vi "Query Element Type.vi"(8 "error in (no error)":errorcluster, 11 "VISA resource name":refnum<visa-resource-name>) -> (0 "error out":errorcluster, 2 "Element Type":i32[](array[numeric]), 3 "VISA resource name out":refnum<visa-resource-name>)   [LabVIEW 2021, in "Yokogawa WT1800 Series.lvlib"]
doc: "Queries the current instrument element type."
uses:
  <instrlib>/Yokogawa WT1800 Series/Yokogawa WT1800 Series.lvlib
panel:
  # "Element 1"
  # "Element 2"
  # "Element 3"
  # "Element 4"
  # "Element 5"
  # "Element 6"
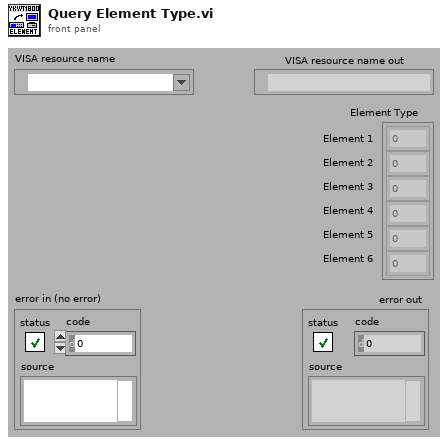
[diagram p1: front panel]
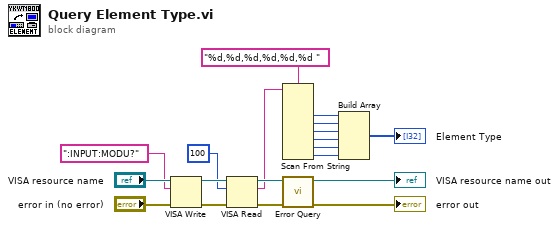
[diagram p0: block diagram]
diagram:
  n1 = VISA Write ("VISA書き込み")(VISA resource name="VISA resource name", write buffer=":INPUT:MODU?" ("書き込みバッファ"), error in (no error)="error in (no error)") -> (VISA resource name out=w19:refnum<visa-resource-name>, error out=w18:errorcluster)  [unwired: 1 out]
  n2 = VISA Read ("VISA読み取り")(VISA resource name=w19, byte count=u32 100, error in (no error)=w18) -> (VISA resource name out=w16:refnum<visa-resource-name>, read buffer=w9:string, error out=w14:errorcluster)  [unwired: 1 out]
  n3 = Scan From String(format string="%d,%d,%d,%d,%d,%d " ("形式文字列"), input string=w9) -> (output 1=w7:i32, output 2=w6:i32, output 3=w5:i32, output 4=w4:i32, output 5=w3:i32, output 6=w2:i32)  [unwired: 8 in, 3 out]
  n4 = call <instrlib>:"Error Query.vi"("error in (no error)"=w14, "VISA resource name"=w16) -> ("error out"=→"error out":errorcluster, "VISA resource name out"=→"VISA resource name out":refnum<visa-resource-name>)  [unwired: 6 in, 2 out]
  n5 = Build Array(w7, w6, w5, w4, w3, w2) -> (→"Element Type":i32[])
